vi "_play_wave_file.vi"(9 "sound length (ms)":dbl, 10 "sound file":path, 11 "sound port":tag="Dev1/ao3") -> ()   [LabVIEW 2024]
uses:
  <vilib>/DAQmx/write.llb/DAQmx Write (Analog 1D Wfm NChan NSamp).vi
  <vilib>/DAQmx/create/channels.llb/DAQmx Create Channel (AO-Voltage-Basic).vi
  <vilib>/sound2/lvsound2.llb/Sound File Info (path).vi
  <vilib>/DAQmx/configure/timing.llb/DAQmx Timing (Sample Clock).vi
  <vilib>/sound2/lvsound2.llb/Sound File Read Open.vi
  <vilib>/sound2/lvsound2.llb/Sound File Read (DBL).vi
  <vilib>/DAQmx/miscellaneous.llb/DAQmx Fill In Error Info.vi
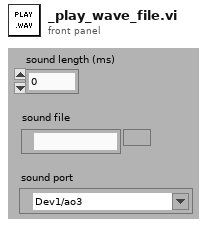
[diagram p1: front panel]
types:
  T1 = typedef "Sound Data Format.ctl" = cluster{"sample rate (S/s)":dbl, "number of channels":i32, "bits per sample":i32}
  T2 = typedef "Sound File Refnum.ctl" = refnum<file>
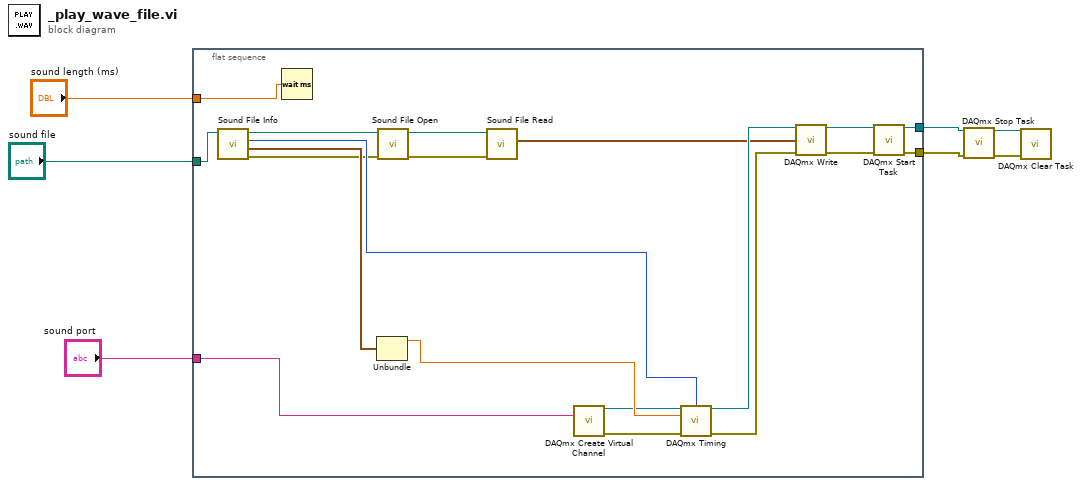
[diagram p0: block diagram]
diagram:
  n1 = flat-sequence {
    tunnel: [w12] -> w7
    tunnel: [w11] -> w6
    tunnel: "sound length (ms)" -> [w10]
    tunnel: "sound file" -> [w9]
    tunnel: "sound port" -> [w8]
    frame #0 {
      n2 = call-poly <vilib>:"Sound File Info.vi"("path"=w9) -> ("error out"=w15:errorcluster, "sound format"=w21:T1, "total number of samples/ch"=w24:u32, "path out"=w14:path)  [unwired: 7 in]
      n3 = Wait (ms)(milliseconds to wait=w10) -> ()  [unwired: 1 out]
      n4 = Unbundle(w21) -> ("sample rate (S/s)"=w23:dbl)  [unwired: 2 out]
      n5 = call-poly <vilib>:"Sound File Open.vi"("error in (no error)"=w15, "path"=w14) -> ("error out"=w16:errorcluster, "sound file refnum"=w13:T2)  [unwired: 8 in]
      n6 = call-poly <vilib>:"Sound File Read.vi"("error in (no error)"=w16, "sound file refnum"=w13) -> ("data"=w25:waveform(dbl)[])  [unwired: 5 in, 4 out]
      n7 = call-poly <vilib>:"DAQmx Create Virtual Channel.vi"("physical channels"=w8) -> ("task out"=w22:refnum<k21>, "error out"=w17:errorcluster)  [unwired: 13 in]
      n8 = call-poly <vilib>:"DAQmx Timing.vi"("task/channels in"=w22, "samples per channel"=w24, "rate"=w23, "error in"=w17) -> ("task out"=w26:refnum<k21>, "error out"=w18:errorcluster)  [unwired: 10 in]
      n9 = call-poly <vilib>:"DAQmx Write.vi"("task/channels in"=w26, "data"=w25, "error in"=w18) -> ("task out"=w20:refnum<k21>, "error out"=w19:errorcluster)  [unwired: 10 in, 1 out]
      n10 = call <vilib>:"DAQmx Start Task.vi"("task/channels in"=w20, "error in"=w19) -> ("task out"=w12:refnum<k21>, "error out"=w11:errorcluster)  [unwired: 12 in]
    }
  }
  n11 = call <vilib>:"DAQmx Stop Task.vi"("task/channels in"=w7, "error in"=w6) -> ("task out"=w2:refnum<k21>, "error out"=w1:errorcluster)  [unwired: 12 in]
  n12 = call <vilib>:"DAQmx Clear Task.vi"("task in"=w2, "error in"=w1) -> ()  [unwired: 13 in, 1 out]
